vi "tcp_query.vi"(7 "response?":bool=TRUE, 8 "error in (no error)":errorcluster, 9 "Termination character":string="\n", 10 "Query String":string, 11 "TCP Network Connection in":refnum<k5>) -> (0 "error out":errorcluster, 2 "Message data out":string, 3 "TCP Network Connection out":refnum<k5>)   [LabVIEW 2025]
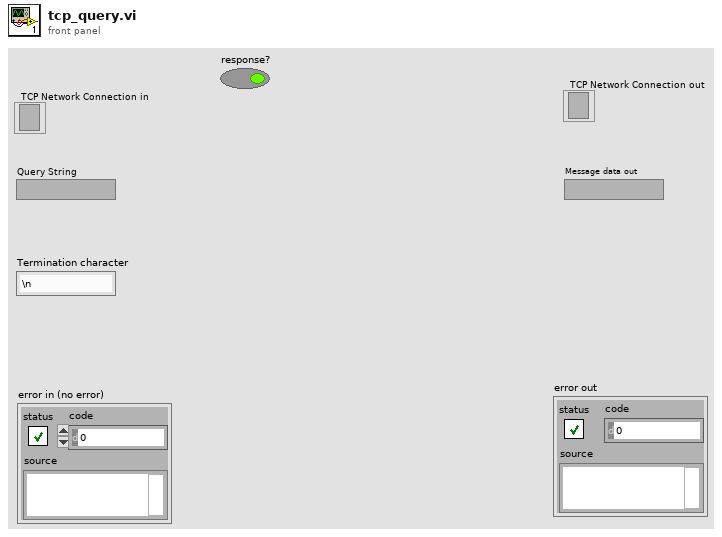
[diagram p1: front panel]
types:
  T1 = enum16{"Standard", "Buffered", "CRLF", "Immediate"}
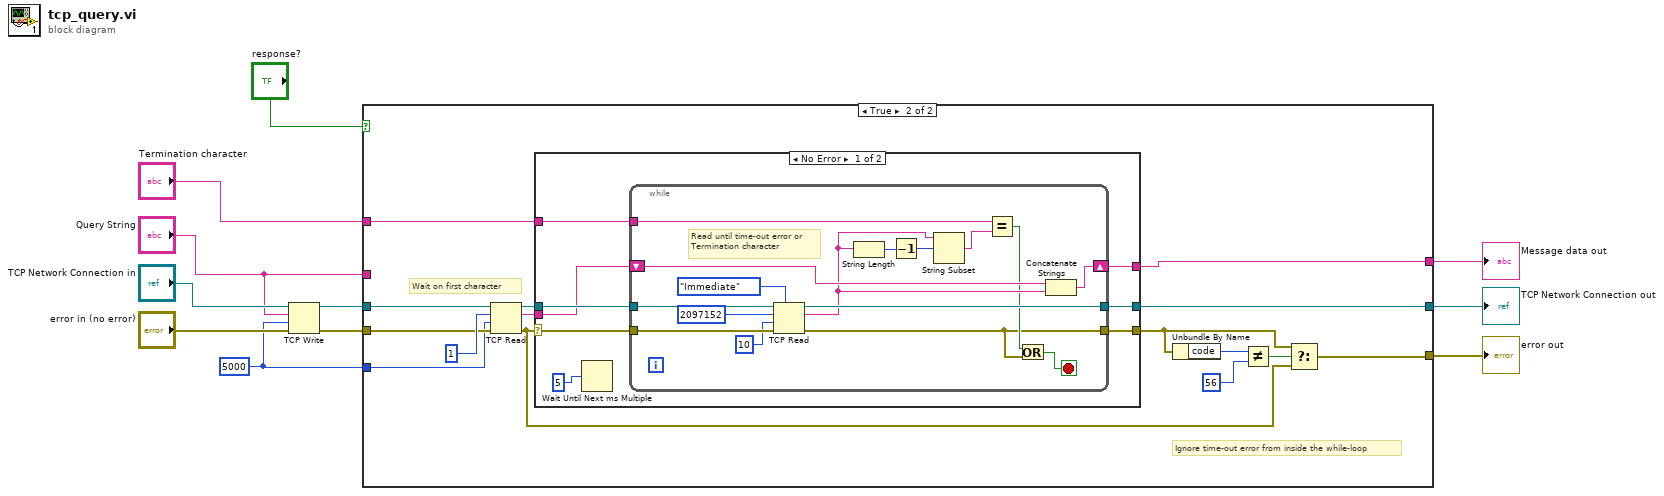
[diagram p0: block diagram]
diagram:
  w5 = 5000 ("timeout ms (25000)")
  n1 = TCP Write(connection ID="TCP Network Connection in", data in="Query String", error in (no error)="error in (no error)", 9:w5) -> (connection ID out=w7:refnum<k5>, error out=w8:errorcluster)  [unwired: 1 out]
  n2 = case shown="True" "response?" {
    tunnel: [w13 w29] -> w11
    tunnel: w8 -> [w12 w27]
    tunnel: w7 -> [w13 w26]
    tunnel: [w14 w23] -> w6
    tunnel: w5 -> [_ w22]
    tunnel: [w12 w18] -> w4
    tunnel: "Termination character" -> [_ w15]
    tunnel: "Query String" -> [w14 _]
    frame False {
    }
    frame True {
      # "Ignore time-out error from inside the while-loop"
      # "Wait on first character"
      n3 = TCP Read(connection ID=w26, bytes to read=1, error in (no error)=w27, 9:w22) -> (connection ID out=w25:refnum<k5>, data out=w24:string, error out=w16:errorcluster)  [unwired: 1 in]
      n4 = case shown="No Error" w16 {
        selector: w16 -> [w32 w54]
        tunnel: [w37 w56] -> w29
        tunnel: [w36 w54] -> w17
        tunnel: w25 -> [w35 w56]
        tunnel: w24 -> [w34 w55]
        tunnel: [w33 w55] -> w23
        tunnel: w15 -> [w30 _]
        frame No Error {
          n5 = Wait Until Next ms Multiple(millisecond multiple=u32 5 ("Milliseconds to Wait (50)")) -> ()  [unwired: 1 out]
          n6 = while {
            tunnel: [w53] -> w37
            tunnel: [w38] -> w36
            tunnel: w35 -> [w51]
            tunnel: w32 -> [w50]
            shift-right: [w47] -> w33
            shift-left: w34 -> [w48]
            tunnel: w30 -> [w41]
            stop <- w40 stop-if-true
            # "Read until time-out error or\nTermination character"
            n7 = TCP Read(connection ID=w51, bytes to read=2097152, error in (no error)=w50, 7:T1."Immediate" ("mode (standard)"), 9:10 ("timeout ms (25000)")) -> (connection ID out=w53:refnum<k5>, data out=w43:string, error out=w38:errorcluster)
            n8 = String Length(string=w43) -> (length=w45:i32)
            n9 = Decrement(x=w45) -> (x-1=w44:i32)
            n10 = String Subset(string=w43, offset (0)=w44) -> (substring=w42:string)  [unwired: 1 in]
            n11 = Equal?(x=w41, y=w42) -> (x = y?=w39:bool)
            n12 = Or(x=w39, y=w38) -> (x .or. y?=w40:bool)
            n13 = Concatenate Strings(w48, w43) -> (w47:string)
          }
        }
        frame Error {
        }
      }
      n14 = Unbundle By Name(w17) -> ("code"=w21:i32)
      n15 = Not Equal?(x=w21, y=56) -> (x != y?=w19:bool)
      n16 = Select(t=w17, s=w19, f=w16) -> (s? t:f=w18:errorcluster)
    }
  }
  "Message data out" <- w6
  "TCP Network Connection out" <- w11
  "error out" <- w4
